vi "Prax12.3.2.vi"(10 "Array":dbl[][](array[numeric])) -> (2 "transposed array":dbl[][](array[numeric]))   [LabVIEW 2020]
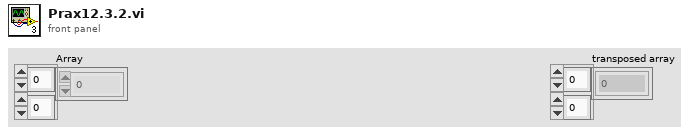
[diagram p1: front panel]
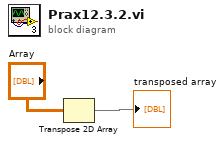
[diagram p0: block diagram]
diagram:
  n1 = Transpose 2D Array(2D array="Array") -> (transposed array=→"transposed array":dbl[][])
